vi "BonOMM-SAOMM.vi"() -> ()   [LabVIEW 2019] (continued)
                          frame True {
                            n3695 = Delete From Array(array=w2986, index=0 ("indice")) -> (deleted portion=w2987:string, array with subset deleted=w2985:string[])  [unwired: 1 in]
                            n3696 = case shown="\"MOVE\"" w2987 {
                              tunnel: w2985 -> [_ _ _]
                              frame "", Default {
                              }
                              frame "MOVE" {
                              }
                              frame "STOP" {
                              }
                            }
                          }
                        }
                      }
                      frame "EINF" {
                        n3697 = Decimal String To Number(string=w2990) -> (number=w2991:i32)  [unwired: 2 in, 1 out]
                        n3698 = case shown="1" w2991 {
                          tunnel: [w2995 w3015 "" w3023] -> w2989
                          frame 0, Default {
                            w2996 = "\n"
                            n3699 = Get Date/Time In Seconds() -> (seconds since 1Jan1904=w2994:timestamp)
                            n3700 = local read "Q String"() -> (w2997:string)
                            n3701 = To Double Precision Float(number=w2994) -> (double precision float=w3000:dbl)
                            n3702 = Get Date/Time String(seconds (now)=w3000, want seconds? (F)=TRUE) -> (date string=w2999:string, time string=w2998:string)  [unwired: 1 in]
                            n3703 = Concatenate Strings(w2999, w2996, w2998, w2996, w2997, w2996, "") -> (w2995:string)
                          }
                          frame 1 {
                            w3017 = "Ferme ta yeule, va t'en chez vous! -> "
                            n3704 = local read "Q String"() -> (w3009:string)
                            n3705 = Random Number (0-1)() -> (number: 0 to 1=w3012:dbl)
                            n3706 = Number To Fractional String(number=w3012, precision (6)=i16 12) -> (F-format string=w3010:string)  [unwired: 2 in]
                            n3707 = String Length(string=w3017) -> (length=w3020:i32)
                            n3708 = Number To Decimal String(number=w3020, width (-)=i16 8) -> (decimal integer string=w3018:string)
                            n3709 = Search and Replace String(replace all?=TRUE ("replace all? (F)"), input string=w3009, search string=",", replace string="\r" ("replace string (\"\")")) -> (result string=w3002:string)  [unwired: 4 in, 3 out]
                            n3710 = Concatenate Strings("ANSW", w3018, w3017, w3010) -> (w3014:string)
                            n3711 = Search and Replace String(replace all?=TRUE ("replace all? (F)"), input string=w3002, search string=";", replace string="\r" ("replace string (\"\")")) -> (result string=w3001:string)  [unwired: 4 in, 3 out]
                            n3712 = Select(t=w3001, s=TRUE, f=w3014) -> (s? t:f=w3015:string)
                          }
                          frame 2 {
                          }
                          frame 3 {
                            n3713 = Get Date/Time In Seconds() -> (seconds since 1Jan1904=w3022:timestamp)
                            n3714 = To Double Precision Float(number=w3022) -> (double precision float=w3027:dbl)
                            n3715 = Get Date/Time String(seconds (now)=w3027) -> (date string=w3026:string, time string=w3025:string)  [unwired: 2 in]
                            n3716 = Concatenate Strings(w3026, "\n", w3025) -> (w3023:string)
                          }
                        }
                        n3717 = local write "ANSW"(w2989) -> ()
                      }
                      frame "ECIB" {
                        # "Commande pour retourner le nom et les coordonnées de la cible"
                        n3718 = Decimal String To Number(string=w3029) -> (number=w3030:i32)  [unwired: 2 in, 1 out]
                        n3719 = case shown="1" w3030 {
                          tunnel: [w3034 w3047 "" w3075] -> w3028
                          frame 0, Default {
                            w3035 = "\n"
                            n3720 = Get Date/Time In Seconds() -> (seconds since 1Jan1904=w3033:timestamp)
                            n3721 = local read "Q String"() -> (w3036:string)
                            n3722 = To Double Precision Float(number=w3033) -> (double precision float=w3039:dbl)
                            n3723 = Get Date/Time String(seconds (now)=w3039, want seconds? (F)=TRUE) -> (date string=w3038:string, time string=w3037:string)  [unwired: 1 in]
                            n3724 = Concatenate Strings(w3038, w3035, w3037, w3035, w3036, w3035, "") -> (w3034:string)
                          }
                          frame 1 {
                            w3046 = "0" ("string")
                            w3050 = "\r" ("replace string (\"\")")
                            w3054 = "\r" ("replace string (\"\")")
                            # "Message d'erreur"
                            # "Message contenant les info de la dernière cible chargées"
                            # "Si la coordonnées de la cible est plus loin de 1 degrés de  celle du télescope, on  envoit un message d'erreur"
                            n3725 = local read "Dec_DC"() -> (w3069:string)
                            n3726 = local read "DEC Tel"() -> (w3067:dbl)
                            n3727 = local read "AD_DC"() -> (w3072:string)
                            n3728 = local read "RA Tel"() -> (w3071:dbl)
                            n3729 = Fract/Exp String To Number(string=w3069) -> (number=w3068:dbl)  [unwired: 3 in, 1 out]
                            n3730 = Fract/Exp String To Number(string=w3072) -> (number=w3070:dbl)  [unwired: 3 in, 1 out]
                            n3731 = Divide(x=w3071, y=3600.0) -> (x/y=w3044:dbl)
                            n3732 = Divide(x=w3067, y=3600.0) -> (x/y=w3043:dbl)
                            n3733 = Subtract(x=w3068, y=w3043) -> (x-y=w3065:dbl)
                            n3734 = Subtract(x=w3070, y=w3044) -> (x-y=w3066:dbl)
                            n3735 = Absolute Value(x=w3065) -> (abs(x)=w3064:dbl)
                            n3736 = Absolute Value(x=w3066) -> (abs(x)=w3063:dbl)
                            n3737 = Greater?(x=w3064, y=1.0) -> (0:w3059:bool)
                            n3738 = Greater?(x=w3063, y=0.067) -> (0:w3060:bool)
                            n3739 = local read "DC_button"() -> (w3057:bool)
                            n3740 = Or(x=w3060, y=w3059) -> (x .or. y?=w3058:bool)
                            n3741 = local read "Numero_DC"() -> (w3056:string)
                            n3742 = local read "Nom_DC"() -> (w3055:string)
                            n3743 = local read "Dec_DC"() -> (w3052:string)
                            n3744 = local read "AD_DC"() -> (w3053:string)
                            n3745 = Or(x=w3058, y=w3057) -> (x .or. y?=w3051:bool)
                            n3746 = Not(x=w3051) -> (.not. x?=w3040:bool)
                            n3747 = Concatenate Strings(w3056, w3054, w3055, w3054, w3053, w3054, w3052) -> (w3048:string)
                            n3748 = Concatenate Strings("-1" ("string"), w3050, w3046, w3050, w3046, w3050, w3046) -> (w3049:string)
                            n3749 = Select(t=w3048, s=w3040, f=w3049) -> (s? t:f=w3047:string)
                            n3750 = local write "DC String"(w3047) -> ()
                          }
                          frame 2 {
                          }
                          frame 3 {
                            n3751 = Get Date/Time In Seconds() -> (seconds since 1Jan1904=w3074:timestamp)
                            n3752 = To Double Precision Float(number=w3074) -> (double precision float=w3079:dbl)
                            n3753 = Get Date/Time String(seconds (now)=w3079) -> (date string=w3078:string, time string=w3077:string)  [unwired: 2 in]
                            n3754 = Concatenate Strings(w3078, "\n", w3077) -> (w3075:string)
                          }
                        }
                        n3755 = local write "ANSW"(w3028) -> ()
                      }
                      frame "EAUT" {
                        n3756 = Decimal String To Number(string=w3081) -> (number=w3080:i32)  [unwired: 2 in, 1 out]
                        n3757 = case shown="1, Par défaut" w3080 {
                          frame 1, Default {
                            n3758 = flat-sequence {
                              tunnel: [w3083] -> w3082
                              tunnel: w3082 -> [w3088]
                              frame #0 {
                                n3759 = Two Button Dialog(message="Donnez vous au gouvernement du Québec\nde négocier un entente de parteneriat association  avec le gouvernement du Canada ? \n", 1:"Non" ("F button name (\"Cancel\")"), 2:"Oui" ("T button name (\"OK\")")) -> (T button?=w3083:bool)
                              }
                              frame #1 {
                                n3760 = case shown="Faux" w3088 {
                                tunnel: ["0" "1"] -> w3087
                                frame False {
                                }
                                frame True {
                                }
                                }
                                n3761 = Concatenate Strings(w3087, "\r") -> (w3089:string)
                                n3762 = local write "ANSW"(w3089) -> ()
                              }
                            }
                          }
                        }
                      }
                      frame "ETMP" {
                        n3763 = Decimal String To Number(string=w3094) -> (number=w3093:i32)  [unwired: 2 in, 1 out]
                        n3764 = case shown="1, Par défaut" w3093 {
                          frame 1, Default {
                            w3108 = "\r"
                            n3765 = local read "indic-T-struct"() -> (w3103:dbl)
                            n3766 = local read "indic-H-out"() -> (w3106:dbl)
                            n3767 = local read "indic-H-in"() -> (w3107:dbl)
                            n3768 = local read "indic-T-out"() -> (w3104:dbl)
                            n3769 = local read "indic-T-in"() -> (w3105:dbl)
                            n3770 = local read "indic-Tm"() -> (w3102:dbl)
                            n3771 = Number To Fractional String(number=w3102) -> (F-format string=w3096:string)  [unwired: 3 in]
                            n3772 = Number To Fractional String(number=w3103) -> (F-format string=w3097:string)  [unwired: 3 in]
                            n3773 = Number To Fractional String(number=w3104) -> (F-format string=w3098:string)  [unwired: 3 in]
                            n3774 = Number To Fractional String(number=w3105) -> (F-format string=w3099:string)  [unwired: 3 in]
                            n3775 = Number To Fractional String(number=w3106) -> (F-format string=w3100:string)  [unwired: 3 in]
                            n3776 = Number To Fractional String(number=w3107) -> (F-format string=w3101:string)  [unwired: 3 in]
                            n3777 = Concatenate Strings(w3101, w3108, w3100, w3108, w3099, w3108, w3098, w3108, w3097, w3108, w3096) -> (w3095:string)
                            n3778 = local write "ANSW"(w3095) -> ()
                          }
                        }
                      }
                      frame "EOFF" {
                        n3779 = call "ETAB_decodeur.vi"("chaine entree"=w3110) -> ("Args"=w3111:string[], "nb args"=w3109:u16)  [unwired: 1 out]
                        n3780 = case shown="3" w3109 {
                          tunnel: w3111 -> [_ w3121 w3284]
                          frame 0, Default {
                          }
                          frame 3 {
                            # "Warning Code"
                            # "Error Code"
                            # "Causait erreur\ncode CYGA à modifier"
                            n3781 = Index Array(array=w3121, index #1=0 ("indice"), index #2=1 ("indice"), index #3=2 ("indice")) -> (element #1=w3112:string, element #2=w3115:string, element #3=w3116:string)
                            n3782 = Fract/Exp String To Number(string=w3116) -> (number=w3113:dbl)  [unwired: 3 in, 1 out]
                            n3783 = Fract/Exp String To Number(string=w3115) -> (number=w3114:dbl)  [unwired: 3 in, 1 out]
                            n3784 = stacked-sequence {
                              seq-local: [_ _ w3206 _ _] -> [_ _ _ w3249 _]
                              seq-local: [_ _ w3231 _ _] -> [_ _ _ w3245 _]
                              seq-local: [_ _ w3230 _ _] -> [_ _ _ w3246 _]
                              tunnel: w3113 -> [w3125 w3146 w3212 _ _]
                              tunnel: w3114 -> [w3134 w3145 w3213 _ _]
                              frame #0 {
                                n3785 = local write "Offset RA"(w3134) -> ()
                                n3786 = Number To Fractional String(number=w3134, precision (6)=i16 2) -> (F-format string=w3129:string)  [unwired: 2 in]
                                n3787 = Number To Fractional String(number=w3125, precision (6)=i16 2) -> (F-format string=w3128:string)  [unwired: 2 in]
                                n3788 = local write "Offset DEC"(w3125) -> ()
                                n3789 = local read "Mode Guidage et Dither"() -> (w3123:bool)
                                n3790 = local read "Guidage en cour"() -> (w3124:bool)
                                n3791 = control-ref of="TERMINAL"() -> (w3136:refnum<vi>)
                                n3792 = control-ref of="Indicateur d'état"() -> (w3135:refnum<vi>)
                                n3793 = Concatenate Strings("Envoi externe d'un offset de " ("string"), w3129, ", " ("string"), w3128) -> (w3127:string)
                                n3794 = And(x=w3124, y=w3123) -> (x .and. y?=w3122:bool)
                                n3795 = call "TERMINAL.vi"("Indicateur Refnum"=w3135, "Terminal Refnum"=w3136, "Indicateur d'état"=w3127) -> ()
                                n3796 = case shown="Vrai" w3122 {
                                frame False {
                                }
                                frame True {
                                # "On désactive le guidage et \non indique au code qu'on guidait avant"
                                n3797 = property on="StopServo" class="Bool (strict)"("Val(Sgnl)"=TRUE ("Value (Signaling)")) -> ()  [unwired: 2 in, 2 out]
                                n3798 = local write "StateGuidageDither"(TRUE ("StateGuidageDither")) -> ()
                                }
                                }
                                n3799 = local write "Offset en cours"(TRUE ("enfoncé")) -> ()
                              }
                              frame #1 {
                                # "Si nous somme en train de guider \nEt que lke mode guidage en dither est activé\nAlors bouge le curseur"
                                # "L'échelle est probablement à revoir,\n c'est le ratio pixel/arcsec"
                                n3800 = local read "StateGuidageDither"() -> (w3140:bool)
                                n3801 = local read "Mode Guidage et Dither"() -> (w3139:bool)
                                n3802 = Divide(x=500.0, y=156.0) -> (x/y=w3144:dbl)
                                n3803 = Multiply(x=w3145, y=w3144) -> (x*y=w3143:dbl)
                                n3804 = And(x=w3140, y=w3139) -> (x .and. y?=w3141:bool)
                                n3805 = Multiply(x=w3144, y=w3146) -> (x*y=w3142:dbl)
                                n3806 = case shown="Vrai" w3141 {
                                tunnel: w3143 -> [_ w3151]
                                tunnel: w3142 -> [_ w3150]
                                frame False {
                                }
                                frame True {
                                # "On bouge le curseur de guide \npour s'ajuster au offset"
                                n3807 = Negate(x=w3150) -> (-x=w3149:dbl)
                                n3808 = local read "XReference"() -> (w3152:dbl)
                                n3809 = local read "YReference"() -> (w3153:dbl)
                                n3810 = control-ref of="ImgArray"() -> (w3156:refnum<vi>)
                                n3811 = local read "ROIHeight"() -> (w3158:u16)
                                n3812 = local read "ROIWidth"() -> (w3157:u16)
                                n3813 = Add(x=w3151, y=w3153) -> (x+y=w3155:dbl)
                                n3814 = Add(x=w3149, y=w3152) -> (x+y=w3154:dbl)
                                n3815 = call "SAOMM-Cursor2ROI.vi"("ImgRef"=w3156, "CursorX"=w3154, "CursorY"=w3155, "ROIWidth"=w3157, "ROIHeight"=w3158) -> ("ROIXOffset"=w3159:u16, "ROIYOffset"=w3160:u16)  [unwired: 7 in, 2 out]
                                n3816 = flat-sequence {
                                tunnel: w3159 -> [w3164]
                                tunnel: w3160 -> [w3163]
                                tunnel: [w3164] -> w3162
                                tunnel: [w3163] -> w3161
                                tunnel: w3162 -> [w3170]
                                tunnel: w3161 -> [w3169]
                                frame #0 {
                                n3817 = local write "ROIXOffset"(w3164) -> ()
                                n3818 = local write "ROIYOffset"(w3163) -> ()
                                }
                                frame #1 {
                                n3819 = local read "Binning"() -> (w3190:u16)
                                n3820 = local read "ROIWidth"() -> (w3184:u16)
                                n3821 = local read "ROIHeight"() -> (w3185:u16)
                                n3822 = local read "Naxis1"() -> (w3188:u16)
                                n3823 = local read "Naxis2"() -> (w3187:u16)
                                n3824 = Bundle("ROIXOffset"=w3170, "ROIYOffset"=w3169) -> (w3186:cluster{"ROIXOffset":u16, "ROIYOffset":u16})  [unwired: 1 in]
                                n3825 = local read "XROIRef"() -> (w3182:dbl)
                                n3826 = Bundle("Naxis1"=w3188, "Naxis2"=w3187) -> (w3189:cluster{"Naxis1":u16, "Naxis2":u16})  [unwired: 1 in]
                                n3827 = Bundle("ROIWidth"=w3184, "ROIHeight"=w3185) -> (w3165:cluster{"ROIWidth":u16, "ROIHeight":u16})  [unwired: 1 in]
                                n3828 = local read "YROIRef"() -> (w3168:dbl)
                                n3829 = Bundle("XROIRef"=w3182, "YROIRef"=w3168) -> (w3183:cluster{"XROIRef":dbl, "YROIRef":dbl})  [unwired: 1 in]
                                n3830 = call "SAOMM-ROI_Fixer.vi"("Binning"=w3190, "Use Offset?"=TRUE, "naxis"=w3189, "ROI"=w3165, "Offset"=w3186, "Reference Pixel"=w3183) -> ("FixedOffset"=w3173:cluster{"ROIXOffset":u16, "ROIYOffset":u16}, "FixedPixel"=w3171:cluster{"PixelX":dbl, "PixelY":dbl})  [unwired: 6 in, 2 out]
                                n3831 = Unbundle By Name(w3173) -> ("ROIXOffset"=w3181:u16, "ROIYOffset"=w3180:u16)
                                n3832 = control-ref of="PrAMS-ACK"() -> (w3193:refnum<vi>)
                                n3833 = local read "MessageType"() -> (w3192:cluster{string[], u32[]})
                                n3834 = control-ref of="PrAMS actif"() -> (w3198:refnum<vi>)
                                n3835 = local read "PrAMS VRN"() -> (w3197:refnum<visa-resource-name>)
                                n3836 = local read "PrAMS Error"() -> (w3196:errorcluster)
                                n3837 = Unbundle By Name(w3171) -> ("PixelX"=w3174:dbl, "PixelY"=w3177:dbl)
                                n3838 = To Double Precision Float(number=w3181) -> (double precision float=w3176:dbl)
                                n3839 = To Double Precision Float(number=w3180) -> (double precision float=w3175:dbl)
                                n3840 = Bundle("ROIYOffset"=w3180, "ROIXOffset"=w3181) -> (w3172:cluster{"ROIYOffset":u16, "ROIXOffset":u16})  [unwired: 1 in]
                                n3841 = Add(x=w3175, y=w3174) -> (x+y=w3167:dbl)
                                n3842 = Add(x=w3176, y=w3177) -> (x+y=w3166:dbl)
                                n3843 = call "SAOMM-UpdateROI.vi"("PRAMMS-COMM IN"=w3197, "Active Refnum"=w3198, "PrAMS-ACK"=w3193, "MessageType"=w3192, "Error IN"=w3196, "Position"=w3172) -> ("PRAMMS-COMM OUT"=w3195:refnum<visa-resource-name>, "Error OUT"=w3194:errorcluster)  [unwired: 7 in, 1 out]
                                n3844 = property on="ImgArray" class="GraphInt (strict)"() -> ("Cursor.Cursor Position"=w3179:T45)  [unwired: 2 in, 2 out]
                                n3845 = local write "XReference"(w3167) -> ()
                                n3846 = local write "YReference"(w3166) -> ()
                                n3847 = local write "PrAMS Error"(w3194) -> ()
                                n3848 = local write "PrAMS VRN"(w3195) -> ()
                                n3849 = Bundle(cluster=w3179, "Cursor X"=w3167, "Cursor Y"=w3166) -> (w3178:T45)
                                n3850 = property on="ImgArray" class="GraphInt (strict)"("Cursor.Cursor Position"=w3178) -> ()  [unwired: 2 in, 2 out]
                                }
                                }
                                }
                                }
                              }
                              frame #2 {
                                w3233 = u32 0 ("Error Code IN")
                                n3851 = control-ref of="Mode"() -> (w3214:refnum<vi>)
                                n3852 = control-ref of="Position Z"() -> (w3220:refnum<vi>)
                                n3853 = control-ref of="DiffX"() -> (w3215:refnum<vi>)
                                n3854 = control-ref of="DiffY"() -> (w3216:refnum<vi>)
                                n3855 = control-ref of="SNR"() -> (w3203:refnum<vi>)
                                n3856 = control-ref of="BrasPesto"() -> (w3199:refnum<vi>)
                                n3857 = control-ref of="MovingXY"() -> (w3202:refnum<vi>)
                                n3858 = local read "Table VRN"() -> (w3224:refnum<visa-resource-name>)
                                n3859 = local read "TCS VRN"() -> (w3226:refnum<visa-resource-name>)
                                n3860 = local read "Table Error"() -> (w3223:errorcluster)
                                n3861 = control-ref of="TCS actif"() -> (w3222:refnum<vi>)
                                n3862 = control-ref of="Table actif"() -> (w3221:refnum<vi>)
                                n3863 = control-ref of="StartServo"() -> (w3219:refnum<vi>)
                                n3864 = control-ref of="Servo"() -> (w3218:refnum<vi>)
                                n3865 = control-ref of="StopServo"() -> (w3217:refnum<vi>)
                                n3866 = local read "TCS Error"() -> (w3225:errorcluster)
                                n3867 = control-ref of="LimXPesto"() -> (w3200:refnum<vi>)
                                n3868 = local read "TableAstrom"() -> (w3227:T4)
                                n3869 = local read "FieldAstrom"() -> (w3229:T4)
                                n3870 = local read "GuiderAstrom"() -> (w3228:T4)
                                n3871 = Bundle("TCS VRN"=w3226, "TCS Error"=w3225, "Table VRN"=w3224, "Table Error"=w3223) -> (w3211:T42)  [unwired: 1 in]
                                n3872 = Bundle("TableAstrom"=w3227, "FieldAstrom"=w3229, "GuiderAstrom"=w3228) -> (w3210:T41)  [unwired: 1 in]
                                n3873 = Bundle("TCS actif"=w3222, "Table actif"=w3221, "Position Z"=w3220, "StartServo"=w3219, "Mode"=w3214, "Servo"=w3218, "StopServo"=w3217, "DiffX"=w3215, "DiffY"=w3216, "SNR"=w3203, "MovingXY"=w3202, "BrasPesto"=w3199, "LimXPesto"=w3200) -> (w3209:T43)  [unwired: 1 in]
                                n3874 = call "Cheesy_Offset.vi"("Communications_Cluster"=w3211, "Astrom_Cluster"=w3210, "RA offset"=w3213, "DEC offset"=w3212, "VariablesReferences"=w3209, "OffsetAccuracy (pixels)"="OffsetAcc") -> ("Error code"=w3208:u8, "Undo offset"=w3206:bool, "Warning code"=w3207:u8, "Error Comment"=w3204:string)  [unwired: 6 in]
                                n3875 = while {
                                tunnel: [FALSE] -> w3201
                                stop <- w3240 continue-if-true
                                n3876 = local read "enfoncé"() -> (w3242:bool)
                                n3877 = Not(x=w3242) -> (.not. x?=w3241:bool)
                                n3878 = Wait (ms)(milliseconds to wait=u32 200) -> ()  [unwired: 1 out]
                                n3879 = local write "enfoncé"(w3241) -> ()
                                n3880 = local read "Offset en cours"() -> (w3240:bool)
                                }
                                n3881 = To Unsigned Long Integer(number=w3208) -> (unsigned 32bit integer=w3230:u32)
                                n3882 = To Unsigned Long Integer(number=w3207) -> (unsigned 32bit integer=w3231:u32)
                                n3883 = local read "FIFO d'erreur"() -> (w3234:T7)
                                n3884 = call "Error_Format.vi"("FIFO IN"=w3234, "Error Code IN"=w3233, "Warning Code IN"=w3233, "Error Bit"=w3230, "Warning Bit"=w3231, "Source"="offset", "Comment"=w3204) -> ("FIFO OUT"=w3235:T7)  [unwired: 10 in, 2 out]
                                n3885 = flat-sequence {
                                tunnel: w3235 -> [w3236]
                                frame #0 {
                                n3886 = local write "FIFO d'erreur"(w3236) -> ()
                                }
                                frame #1 {
                                n3887 = local write "Offset en cours"(FALSE) -> ()
                                }
                                }
                                n3888 = local write "enfoncé"(w3201) -> ()
                              }
                              frame #3 {
                                w3251 = FALSE
                                w3244 = FALSE
                                # "Préparation de la réponse ..."
                                n3889 = local write "Offset OK"(w3244) -> ()
                                n3890 = local write "TCS actif"(w3244) -> ()
                                n3891 = local write "RangeTable"(w3251) -> ()
                                n3892 = local write "Calibration"(w3251) -> ()
                                n3893 = local write "stoptable"(w3251) -> ()
                                n3894 = local write "Alacible"(w3251) -> ()
                                n3895 = local write "Origine"(w3251) -> ()
                                n3896 = local write "Centre"(w3251) -> ()
                                n3897 = local read "TERMINAL"() -> (w3255:string)
                                n3898 = Greater Than 0?(x=w3246) -> (x > 0?=w3247:bool)
                                n3899 = case shown="Vrai" w3247 {
                                tunnel: [w3258 w3262] -> w3248
                                tunnel: w3246 -> [_ w3261]
                                tunnel: w3245 -> [w3257 _]
                                frame False {
                                n3900 = Number To Decimal String(number=w3257) -> (decimal integer string=w3260:string)  [unwired: 1 in]
                                n3901 = Concatenate Strings("W" ("string"), w3260) -> (w3258:string)
                                }
                                frame True {
                                n3902 = Number To Decimal String(number=w3261) -> (decimal integer string=w3264:string)  [unwired: 1 in]
                                n3903 = Concatenate Strings("E" ("string"), w3264) -> (w3262:string)
                                }
                                }
                                n3904 = Select(t=" : échoué" ("Command String"), s=w3249, f=" : réussi" ("Command String")) -> (s? t:f=w3256:string)
                                n3905 = Concatenate Strings(w3255, w3256) -> (w3254:string)
                                n3906 = local write "TERMINAL"(w3254) -> ()
                                n3907 = Select(t=w3248, s=w3249, f="OK" ("Command String")) -> (s? t:f=w3243:string)
                                n3908 = local write "ANSW"(w3243) -> ()
                                n3909 = case shown="Vrai" w3249 {
                                frame False {
                                }
                                frame True {
                                n3910 = local read "Table VRN"() -> (w3269:refnum<visa-resource-name>)
                                n3911 = control-ref of="Table actif"() -> (w3267:refnum<vi>)
                                n3912 = local read "Table Error"() -> (w3266:errorcluster)
                                n3913 = control-ref of="TCS actif"() -> (w3270:refnum<vi>)
                                n3914 = local read "TCS VRN"() -> (w3271:refnum<visa-resource-name>)
                                n3915 = call "EXCOM-CMD.vi"("VRN IN"=w3271, "Bool Refnum"=w3270, "Commande #"=13) -> ("VRN OUT"=w3272:refnum<visa-resource-name>, "Error OUT"=w3273:errorcluster)  [unwired: 10 in, 1 out]
                                n3916 = call "Newmark-Stop.vi"("Table VRN IN"=w3269, "Bool Refnum"=w3267, "Error IN"=w3266) -> ("Table VRN OUT"=w3268:refnum<visa-resource-name>, "Error OUT"=w3265:errorcluster)  [unwired: 11 in]
                                n3917 = local write "Table Error"(w3265) -> ()
                                n3918 = local write "Table VRN"(w3268) -> ()
                                n3919 = local write "TCS VRN"(w3272) -> ()
                                n3920 = local write "TCS Error"(w3273) -> ()
                                }
                                }
                              }
                              frame #4 {
                                # "Si le mode de guidage est activé \net qu'on guidait avant"
                                n3921 = local read "StateGuidageDither"() -> (w3275:bool)
                                n3922 = local read "Mode Guidage et Dither"() -> (w3276:bool)
                                n3923 = And(x=w3275, y=w3276) -> (x .and. y?=w3277:bool)
                                n3924 = case shown="Vrai" w3277 {
                                frame False {
                                }
                                frame True {
                                # "Réactive le guidage\nMet la variable de retenir qu'on guidait à off"
                                n3925 = local write "StateGuidageDither"(FALSE ("StateGuidageDither")) -> ()
                                n3926 = property on="StartServo" class="Bool (strict)"("Val(Sgnl)"=TRUE ("Value (Signaling)")) -> ()  [unwired: 2 in, 2 out]
                                }
                                }
                              }
                            }
                            n3927 = Not Equal?(x=w3112, y="N") -> ()  [unwired: 1 out]
                          }
                          frame 4 {
                            # "Lorsqu'il y a un argument additionnel a teloffset."
                            n3928 = Index Array(array=w3284, index #1=0 ("indice"), index #2=1 ("indice"), index #3=2 ("indice"), index #4=3 ("index")) -> (element #1=w3285:string, element #2=w3286:string, element #3=w3287:string, element #4=w3280:string)
                            n3929 = Fract/Exp String To Number(string=w3287) -> (number=w3282:dbl)  [unwired: 3 in, 1 out]
                            n3930 = Fract/Exp String To Number(string=w3286) -> (number=w3283:dbl)  [unwired: 3 in, 1 out]
                            n3931 = Not Equal?(x=w3285, y="N") -> ()  [unwired: 1 out]
                            n3932 = case shown="\"T\"" w3280 {
                              tunnel: w3283 -> [_ w3293]
                              tunnel: w3282 -> [_ w3292]
                              frame "False", Default {
                              }
                              frame "T" {
                                # "Teloffset à l'aide de la télécommande du télescope"
                                n3933 = local write "GE_TCS_RA"(w3293) -> ()
                                n3934 = local write "GE_TCS_DEC"(w3292) -> ()
                              }
                            }
                          }
                        }
                      }
                      frame "ELIB" {
                      }
                      frame "ERAF" {
                        n3935 = call "ETAB_decodeur.vi"("chaine entree"=w3295) -> ("Args"=w3298:string[])  [unwired: 2 out]
                        n3936 = Index Array(array=w3298) -> (element=w3297:string)  [unwired: 1 in]
                        n3937 = local read "MC-BonOMM VRN"() -> (w3296:refnum<visa-resource-name>)
                        n3938 = local read "Excmd VRN"() -> (w3294:refnum<visa-resource-name>)
                        n3939 = case shown="\"i\"" w3297 {
                          selector: w3297 -> [_ _ _ w3337 _]
                          tunnel: w3296 -> [_ w3304 w3320 _ _]
                          tunnel: w3294 -> [_ w3299 w3315 w3334 w3363]
                          frame "", Default {
                          }
                          frame "m" {
                            n3940 = call "MC-BonOMM_talker.vi"("MC-BonOMM VRN"=w3304, "Commande"="m", "byte count"=u32 1, "answer=command?"=FALSE) -> ("Answer"=w3301:string, "ok ?"=w3300:bool)  [unwired: 1 in]
                            n3941 = case shown="Vrai" w3300 {
                              tunnel: w3301 -> [_ w3307]
                              tunnel: w3299 -> [_ w3312]
                              frame False {
                              }
                              frame True {
                                n3942 = Concatenate Strings(w3307, "\n" ("string")) -> (w3306:string)
                                n3943 = String Length(string=w3306) -> (length=w3314:i32)
                                n3944 = Number To Decimal String(number=w3314, width (-)=i16 4 ("largeur (-)")) -> (decimal integer string=w3310:string)
                                n3945 = Concatenate Strings("ANSW", w3310, w3306) -> (w3309:string)
                                n3946 = VISA Write(VISA resource name=w3312, write buffer=w3309) -> ()  [unwired: 1 in, 3 out]
                              }
                            }
                          }
                          frame "q" {
                            n3947 = call "MC-BonOMM_talker.vi"("MC-BonOMM VRN"=w3320, "Commande"="q", "byte count"=u32 1, "answer=command?"=FALSE) -> ("Answer"=w3317:string, "ok ?"=w3316:bool)  [unwired: 1 in]
                            n3948 = case shown="Vrai" w3316 {
                              tunnel: w3317 -> [_ w3324]
                              tunnel: w3315 -> [_ w3328]
                              frame False {
                              }
                              frame True {
                                n3949 = Concatenate Strings(w3324, "\n" ("string")) -> (w3322:string)
                                n3950 = String Length(string=w3322) -> (length=w3330:i32)
                                n3951 = Number To Decimal String(number=w3330, width (-)=i16 4 ("largeur (-)")) -> (decimal integer string=w3326:string)
                                n3952 = Concatenate Strings("ANSW", w3326, w3322) -> (w3325:string)
                                n3953 = VISA Write(VISA resource name=w3328, write buffer=w3325) -> ()  [unwired: 1 in, 3 out]
                              }
                            }
                          }
                          frame "1", "2", "3", "4", "5", "6" {
                            n3954 = Decimal String To Number(string=w3337) -> (number=w3338:i32)  [unwired: 2 in, 1 out]
                            n3955 = case shown="6" w3338 {
                              frame 0, Default {
                              }
                              frame 1 {
                                n3956 = property on="filtre #1" class="Bool (strict)"("Value (Signaling)"=TRUE) -> ()  [unwired: 2 in, 2 out]
                              }
                              frame 2 {
                                n3957 = property on="filtre #2" class="Bool (strict)"("Value (Signaling)"=TRUE) -> ()  [unwired: 2 in, 2 out]
                              }
                              frame 3 {
                                n3958 = property on="filtre #3" class="Bool (strict)"("Value (Signaling)"=TRUE) -> ()  [unwired: 2 in, 2 out]
                              }
                              frame 4 {
                                n3959 = property on="filtre #4" class="Bool (strict)"("Value (Signaling)"=TRUE) -> ()  [unwired: 2 in, 2 out]
                              }
                              frame 5 {
                                n3960 = property on="filtre #5" class="Bool (strict)"("Value (Signaling)"=TRUE) -> ()  [unwired: 2 in, 2 out]
                              }
                              frame 6 {
                                n3961 = property on="filtre #6" class="Bool (strict)"("Value (Signaling)"=TRUE) -> ()  [unwired: 2 in, 2 out]
                              }
                            }
                            n3962 = while {
                              tunnel: w3334 -> [_]
                              tunnel: w3338 -> [w3361]
                              tunnel: [FALSE ("Bypass Tech")] -> w3335
                              tunnel: [w3355] -> w3332
                              tunnel: [w3354] -> w3331
                              i -> [w3359]
                              stop <- w3360 stop-if-true
                              n3963 = local read "F#"() -> (w3355:i32)
                              n3964 = Wait (ms)(milliseconds to wait=u32 200) -> ()  [unwired: 1 out]
                              n3965 = Equal?(x=w3355, y=w3361) -> (x = y?=w3354:bool)
                              n3966 = call "Max-iteration.vi"("i max"=150, "i act"=w3359, "Valeur entrante"=w3354) -> ("break ?"=w3360:bool)
                            }
                            n3967 = Number To Decimal String(number=w3332) -> (decimal integer string=w3333:string)  [unwired: 1 in]
                            n3968 = case shown="Faux" w3331 {
                              tunnel: w3334 -> [_ w3345]
                              tunnel: w3333 -> [_ w3339]
                              frame False {
                              }
                              frame True {
                                n3969 = Concatenate Strings(w3339, "\n" ("string")) -> (w3340:string)
                                n3970 = String Length(string=w3340) -> (length=w3347:i32)
                                n3971 = Number To Decimal String(number=w3347, width (-)=i16 4 ("largeur (-)")) -> (decimal integer string=w3343:string)
                                n3972 = Concatenate Strings("ANSW", w3343, w3340) -> (w3342:string)
                                n3973 = VISA Write(VISA resource name=w3345, write buffer=w3342) -> ()  [unwired: 1 in, 3 out]
                              }
                            }
                            n3974 = local write "Bypass Tech"(w3335) -> ()
                            "Bypass Tech" <- TRUE ("Bypass Tech")
                          }
                          frame "i" {
                            n3975 = local read "Tableau des filtres"() -> (w3370:string[])
                            n3976 = local write "string temporaire"("") -> ()
                            n3977 = for {
                              tunnel: w3370 -> [w3374] mode=indexing
                              tunnel: [w3371] -> w3362
                              n3978 = Concatenate Strings("string temporaire", w3374, "\n" ("string")) -> (w3371:string)
                              n3979 = local write "string temporaire"(w3371) -> ()
                            }
                            n3980 = String Length(string=w3362) -> (length=w3368:i32)
                            n3981 = Number To Decimal String(number=w3368, width (-)=i16 4 ("largeur (-)")) -> (decimal integer string=w3365:string)
                            n3982 = Concatenate Strings("ANSW", w3365, w3362) -> (w3364:string)
                            n3983 = VISA Write(VISA resource name=w3363, write buffer=w3364) -> ()  [unwired: 1 in, 3 out]
                          }
                        }
                      }
                      frame "EHEX" {
                      }
                    }
                  }
                  frame #1 {
                    # "Envoie la réponse sur le port approprié"
                    n3984 = String Subset(string=w3376, length (rest)=3 ("length (rest)")) -> (substring=w3378:string)  [unwired: 1 in]
                    n3985 = Equal?(x=w3378, y="COM") -> (x = y?=w3377:bool)
                    n3986 = case shown="Faux" w3377 {
                      tunnel: w3376 -> [w3391 w3403]
                      tunnel: "ANSW" -> [w3383 w3395]
                      frame False {
                        # "Réponse TCP/IP"
                        n3987 = Type Cast(type=refnum<k5> refnum ("connection ID out"), x=w3391) -> (*(type *) &x=w3390:refnum<k5>)
                        n3988 = String Length(string=w3383) -> (length=w3387:i32)
                        n3989 = Number To Decimal String(number=w3387, width (-)=i16 8) -> (decimal integer string=w3385:string)
                        n3990 = Concatenate Strings("ANSW", w3385, w3383) -> (w3382:string)
                        n3991 = TCP Write(connection ID=w3390, data in=w3382, 9:500 ("timeout ms (25000)")) -> (error out=w3388:errorcluster)  [unwired: 1 in, 2 out]
                        n3992 = local write "TCP/IP Error"(w3388) -> ()
                      }
                      frame True {
                        # "Réponse sur le port Série ..."
                        n3993 = local read "Excmd VRN"() -> (w3404:refnum<visa-resource-name>)
                        n3994 = Type Cast(type=w3404, x=w3403) -> (*(type *) &x=w3402:refnum<visa-resource-name>)
                        n3995 = Concatenate Strings(w3395, "\n") -> (w3396:string)
                        n3996 = String Length(string=w3396) -> (length=w3400:i32)
                        n3997 = Number To Decimal String(number=w3400, width (-)=i16 4) -> (decimal integer string=w3399:string)
                        n3998 = Concatenate Strings("ANSW", w3399, w3396) -> (w3397:string)
                        n3999 = local read "Excom Error"() -> (w3393:errorcluster)
                        n4000 = VISA Write(VISA resource name=w3402, write buffer=w3397, error in (no error)=w3393) -> (error out=w3392:errorcluster)  [unwired: 2 out]
                        n4001 = local write "Excom Error"(w3392) -> ()
                      }
                    }
                  }
                }
                "Error Code" <- w2858
                "Warning Code" <- w2858
              }
            }
            n4002 = Wait Until Next ms Multiple(millisecond multiple=u32 50 ("n millisecondes")) -> ()  [unwired: 1 out]
            n4003 = local read "Quit"() -> (w2851:bool)
          }
          "Gestion Scripts" <- w970
          n4004 = while {
            tunnel: [w1440] -> w975
            i -> [w1441]
            stop <- w1440 stop-if-true
            n4005 = event shown="[0] Timeout" {
              selector: _ -> [_ _ _ _ _ _ _ _ _ _ _ _ _ _ _ _ _ _ _ _ _ _ _]
              dyn-events: _ -> [_ _ _ _ _ _ _ _ _ _ _ _ _ _ _ _ _ _ _ _ _ _ _]
              timeout: 200 -> [_ _ _ _ _ _ _ _ _ _ _ _ _ _ _ _ _ _ _ _ _ _ _]
              tunnel: w1441 -> [w1449 _ _ _ _ _ _ _ _ _ _ _ _ _ _ _ _ _ _ _ _ _ _]
              event Timeout {
                # "À passer dans une boucle à part ?"
                n4006 = event-data() -> ()  [unwired: 1 in, 2 out]
                n4007 = local read "Integrating"() -> (w1446:bool)
                n4008 = Quotient & Remainder(x=w1449, y=25) -> (x-y*floor(x/y)=w1447:i32)  [unwired: 1 out]
                n4009 = Equal To 0?(x=w1449) -> (x = 0?=w1451:bool)
                n4010 = Equal To 0?(x=w1447) -> (x = 0?=w1445:bool)
                n4011 = Not(x=w1446) -> (.not. x?=w1444:bool)
                n4012 = And(x=w1445, y=w1444) -> (x .and. y?=w1443:bool)
                n4013 = Or(x="FalconRefresh", y=w1451) -> (x .or. y?=w1456:bool)
                n4014 = Equal?(x=w1449, y=1) -> (x = y?=w1453:bool)
                n4015 = Compound Arithmetic op=OR(w1453, "HexapodRefresh", w1443) -> (w1450:bool)
                n4016 = case shown="Faux" w1456 {
                  frame False {
                  }
                  frame True {
                    n4017 = Tick Count (ms)() -> (millisecond timer value=→"FalconQuery":u32)
                    n4018 = local write "FalconRefresh"(FALSE ("Refresh")) -> ()
                    n4019 = local read "PrAMS VRN"() -> (w1473:refnum<visa-resource-name>)
                    n4020 = local read "PrAMS Error"() -> (w1475:errorcluster)
                    n4021 = local read "MessageType"() -> (w1470:cluster{string[], u32[]})
                    n4022 = control-ref of="PrAMS actif"() -> (w1471:refnum<vi>)
                    n4023 = local read "Signature"() -> (w1469:u32)
                    n4024 = call "SAOMM-QueryFalcon.vi"("PRAMMS-COMM IN"=w1473, "Bool Refnum"=w1471, "Signature"=w1469, "Error IN"=w1475, "CommandCluster"=w1470) -> ("PRAMMS-COMM OUT"=w1472:refnum<visa-resource-name>, "Error OUT"=w1474:errorcluster)  [unwired: 9 in]
                    n4025 = local write "PrAMS Error"(w1474) -> ()
                    n4026 = local write "PrAMS VRN"(w1472) -> ()
                    "QueryingPraMS" <- TRUE
                  }
                }
                n4027 = case shown="Vrai" w1450 {
                  frame False {
                  }
                  frame True {
                    n4028 = local write "HexapodRefresh"(FALSE ("Refresh")) -> ()
                    n4029 = Tick Count (ms)() -> (millisecond timer value=→"HexapodQuery":u32)
                    n4030 = local read "MessageType"() -> (w1462:cluster{string[], u32[]})
                    n4031 = control-ref of="HexaCons actif"() -> (w1458:refnum<vi>)
                    n4032 = local read "PrAMS Error"() -> (w1464:errorcluster)
                    n4033 = local read "Signature"() -> (w1461:u32)
                    n4034 = call "SAOMM-QueryHexapod.vi"("PRAMMS-COMM IN"="Hexapod VRN", "Bool Refnum"=w1458, "Signature"=w1461, "Error IN"=w1464, "EnumMessageType"=w1462) -> ("PRAMMS-COMM OUT"=w1459:refnum<visa-resource-name>, "Error OUT"=w1463:errorcluster)  [unwired: 9 in]
                    n4035 = local write "PrAMS Error"(w1463) -> ()
                    n4036 = local write "Hexapod VRN"(w1459) -> ()
                    "QueryingHexapod" <- TRUE ("Refresh")
                  }
                }
              }
              event "refresh": Value Change {
                n4037 = event-data() -> ()  [unwired: 1 in, 5 out]
                n4038 = case shown="Vrai" "refresh" {
                  frame False {
                  }
                  frame True {
                    n4039 = flat-sequence {
                      frame #0 {
                        n4040 = local read "MessageType"() -> (w1485:cluster{string[], u32[]})
                        n4041 = control-ref of="PrAMS actif"() -> (w1484:refnum<vi>)
                        n4042 = local read "PrAMS VRN"() -> (w1483:refnum<visa-resource-name>)
                        n4043 = local read "PrAMS Error"() -> (w1482:errorcluster)
                        n4044 = local read "Signature"() -> (w1481:u32)
                        n4045 = call "SAOMM-SendGET.vi"("PRAMMS-COMM IN"=w1483, "Bool Refnum"=w1484, "MessageType"=w1485, "Signature"=w1481, "Error IN"=w1482, "Active GET"="GetCommand") -> ("PRAMMS-COMM OUT"=w1480:refnum<visa-resource-name>, "Error OUT"=w1479:errorcluster)  [unwired: 8 in]
                        n4046 = local write "PrAMS Error"(w1479) -> ()
                        n4047 = local write "PrAMS VRN"(w1480) -> ()
                      }
                      frame #1 {
                        n4048 = local write "refresh"(FALSE) -> ()
                      }
                    }
                  }
                }
              }
              event "Mode": Value Change {
                # "C'est ici qu'on changera les mutex pour les boutons quand ceux-ci seront définis ..."
                n4049 = event-data() -> ("OldVal"=w1488:u16, "NewVal"=w1487:u16)  [unwired: 1 in, 3 out]
                n4050 = case shown="0, Par défaut" w1488 {
                  frame 0, Default {
                    # "On passe de 'Opération fixe' à ..."
                  }
                  frame 1 {
                    # "On passe de 'Asservissement passif' à ..."
                  }
                  frame 2 {
                    # "On passe de 'Asservissement actif' à ..."
                  }
                  frame 3 {
                    # "On passe de 'Calibration' à ..."
                  }
                }
                n4051 = case shown="1..3" w1487 {
                  frame 0, Default {
                    # "... 'Opération fixe'"
                  }
                  frame 4 {
                    w1489 = T17."Enabled" ("Disabled")
                    # "On passe de 'Opération fixe' à ..."
                    n4052 = property on="StartServo" class="Bool (strict)"("DisabledEnum"=w1489) -> ()  [unwired: 2 in, 2 out]
                    n4053 = property on="StopServo" class="Bool (strict)"("DisabledEnum"=w1489) -> ()  [unwired: 2 in, 2 out]
                  }
                  frame 1..3 {
                    # "'Asservissement passif'"
                    n4054 = local read "Integrating"() -> (w1490:bool)
                    n4055 = case shown="Faux" w1490 {
                      frame False {
                        w1491 = T17."Disabled and Grayed Out" ("Disabled")
                        n4056 = property on="StopServo" class="Bool (strict)"("DisabledEnum"=w1491) -> ()  [unwired: 2 in, 2 out]
                        n4057 = property on="StartServo" class="Bool (strict)"("DisabledEnum"=w1491) -> ()  [unwired: 2 in, 2 out]
                      }
                      frame True {
                      }
                    }
                  }
                }
              }
              event "ImgArray": Mouse Down {
                n4058 = event-data() -> ("Coords"=w1496:T50)  [unwired: 1 in, 6 out]
                n4059 = local read "Integrating"() -> (w1494:bool)
                n4060 = local read "Servo"() -> (w1493:bool)
                n4061 = Not(x=w1493) -> (.not. x?=w1492:bool)
                n4062 = And(x=w1494, y=w1492) -> (x .and. y?=w1495:bool)
                n4063 = case shown="Vrai" w1495 {
                  tunnel: w1496 -> [_ w1531]
                  tunnel: w1492 -> [w1497 _]
                  frame False {
                    n4064 = case shown="Faux" w1497 {
                      frame False {
                        n4065 = One Button Dialog(message="Vous ne pouvez pas modifier la ROI pendant l'asservissement") -> ()  [unwired: 1 in, 1 out]
                      }
                      frame True {
                      }
                    }
                  }
                  frame True {
                    n4066 = control-ref of="ImgArray"() -> (w1528:refnum<vi>)
                    n4067 = local read "ROIWidth"() -> (w1527:u16)
                    n4068 = local read "ROIHeight"() -> (w1526:u16)
                    n4069 = call "Click2CursorPosition.vi"("reference"=w1528, "ClickPosition"=w1531) -> ("CursorX"=w1530:dbl, "CursorY"=w1529:dbl)  [unwired: 12 in]
                    n4070 = call "SAOMM-Cursor2ROI.vi"("ImgRef"=w1528, "CursorX"=w1530, "CursorY"=w1529, "ROIWidth"=w1527, "ROIHeight"=w1526) -> ("XÉtoile"=w1504:dbl, "YÉtoile"=w1503:dbl, "ROIXOffset"=w1508:u16, "ROIYOffset"=w1507:u16)  [unwired: 7 in]
                    n4071 = local write "YROIRef"(w1504) -> ()
                    n4072 = local write "XROIRef"(w1503) -> ()
                    n4073 = local write "ROIXOffset"(w1508) -> ()
                    n4074 = local write "ROIYOffset"(w1507) -> ()
                    n4075 = local read "Binning"() -> (w1517:u16)
                    n4076 = local read "ROIWidth"() -> (w1510:u16)
                    n4077 = local read "ROIHeight"() -> (w1511:u16)
                    n4078 = local read "Naxis1"() -> (w1515:u16)
                    n4079 = local read "Naxis2"() -> (w1514:u16)
                    n4080 = Bundle("XÉtoile"=w1504, "YÉtoile"=w1503) -> (w1509:cluster{"XÉtoile":dbl, "YÉtoile":dbl})  [unwired: 1 in]
                    n4081 = Bundle("Naxis1"=w1515, "Naxis2"=w1514) -> (w1516:cluster{"Naxis1":u16, "Naxis2":u16})  [unwired: 1 in]
                    n4082 = Bundle("ROIWidth"=w1510, "ROIHeight"=w1511) -> (w1513:cluster{"ROIWidth":u16, "ROIHeight":u16})  [unwired: 1 in]
                    n4083 = Bundle("ROIXOffset"=w1508, "ROIYOffset"=w1507) -> (w1512:cluster{"ROIXOffset":u16, "ROIYOffset":u16})  [unwired: 1 in]
                    n4084 = control-ref of="PrAMS-ACK"() -> (w1520:refnum<vi>)
                    n4085 = local read "MessageType"() -> (w1519:cluster{string[], u32[]})
                    n4086 = control-ref of="PrAMS actif"() -> (w1525:refnum<vi>)
                    n4087 = local read "PrAMS VRN"() -> (w1524:refnum<visa-resource-name>)
                    n4088 = local read "PrAMS Error"() -> (w1523:errorcluster)
                    n4089 = call "SAOMM-ROI_Fixer.vi"("Binning"=w1517, "Use Offset?"=TRUE, "naxis"=w1516, "ROI"=w1513, "Offset"=w1512, "Reference Pixel"=w1509) -> ("FixedOffset"=w1501:cluster{"ROIXOffset":u16, "ROIYOffset":u16}, "FixedPixel"=w1502:cluster{"PixelX":dbl, "PixelY":dbl})  [unwired: 6 in, 2 out]
                    n4090 = Unbundle By Name(w1502) -> ("PixelX"=w1500:dbl, "PixelY"=w1499:dbl)
                    n4091 = call "SAOMM-UpdateROI.vi"("PRAMMS-COMM IN"=w1524, "Active Refnum"=w1525, "PrAMS-ACK"=w1520, "MessageType"=w1519, "Error IN"=w1523, "Position"=w1501) -> ("PRAMMS-COMM OUT"=w1522:refnum<visa-resource-name>, "Error OUT"=w1521:errorcluster)  [unwired: 7 in, 1 out]
                    n4092 = local write "PrAMS Error"(w1521) -> ()
                    n4093 = local write "PrAMS VRN"(w1522) -> ()
                    n4094 = property on="ImgArray" class="GraphInt (strict)"() -> ("Cursor.Cursor Position"=w1506:T45)  [unwired: 2 in, 2 out]
                    n4095 = local write "XReference"(w1500) -> ()
                    n4096 = local write "YReference"(w1499) -> ()
                    n4097 = Bundle(cluster=w1506, "Cursor X"=w1500, "Cursor Y"=w1499) -> (w1505:T45)
                    n4098 = property on="ImgArray" class="GraphInt (strict)"("Cursor.Cursor Position"=w1505) -> ()  [unwired: 2 in, 2 out]
                  }
                }
              }
              event "ClearDump": Value Change {
                # "Tout ceci est du débuggage ..."
                n4099 = event-data() -> ()  [unwired: 1 in, 5 out]
                n4100 = local write "nDumped"(0 ("nDumped")) -> ()
                n4101 = local write "Dump"("") -> ()
              }
              event "ImageFPS": Value Change {
                n4102 = event-data() -> ()  [unwired: 1 in, 5 out]
                n4103 = flat-sequence {
                  tunnel: [w1536] -> w1535
                  tunnel: [w1539] -> w1534
                  tunnel: w1535 -> [w1539]
                  tunnel: w1534 -> [w1551]
                  frame #0 {
                    n4104 = Tick Count (ms)() -> (millisecond timer value=w1536:u32)
                  }
                  frame #1 {
                    n4105 = local read "MessageType"() -> (w1542:cluster{string[], u32[]})
                    n4106 = control-ref of="PrAMS-ACK"() -> (w1543:refnum<vi>)
                    n4107 = control-ref of="PrAMS actif"() -> (w1544:refnum<vi>)
                    n4108 = local read "PrAMS Error"() -> (w1545:errorcluster)
                    n4109 = local read "PrAMS VRN"() -> (w1546:refnum<visa-resource-name>)
                    n4110 = local read "ImageFPS"() -> (w1537:dbl)
                    n4111 = local read "Signature"() -> (w1538:u32)
                    n4112 = call-poly "SAOMM-Num2littleEndian.vi"("Number"=w1537) -> ("LiitleEndianedData"=w1540:u8[])  [unwired: 14 in]
                    n4113 = call "SAOMM-SendSET.vi"("PRAMMS-COMM IN"=w1546, "Active Refnum"=w1544, "PrAMS-ACK"=w1543, "Signature"=w1538, "Error IN"=w1545, "MessageType"=w1542, "Active SET"="emtSetImageDisplayFrameRate", "Value (little endianed byte array)"=w1540) -> ("PRAMMS-COMM OUT"=w1548:refnum<visa-resource-name>, "Error OUT"=w1547:errorcluster)  [unwired: 4 in, 2 out]
                    n4114 = local write "PrAMS Error"(w1547) -> ()
                    n4115 = local write "PrAMS VRN"(w1548) -> ()
                  }
                  frame #2 {
                    n4116 = Tick Count (ms)() -> (millisecond timer value=w1550:u32)
                    n4117 = Subtract(x=w1550, y=w1551) -> (x-y=→"SetFPSTime":u32)
                  }
                }
              }
              event "exptime": Value Change {
                n4118 = event-data() -> ()  [unwired: 1 in, 5 out]
                n4119 = flat-sequence {
                  tunnel: [w1554] -> w1553
                  tunnel: [w1556] -> w1552
                  tunnel: w1553 -> [w1556]
                  tunnel: w1552 -> [w1571]
                  frame #0 {
                    n4120 = Tick Count (ms)() -> (millisecond timer value=w1554:u32)
                  }
                  frame #1 {
                    n4121 = local read "MessageType"() -> (w1562:cluster{string[], u32[]})
                    n4122 = control-ref of="PrAMS-ACK"() -> (w1563:refnum<vi>)
                    n4123 = control-ref of="PrAMS actif"() -> (w1564:refnum<vi>)
                    n4124 = local read "PrAMS Error"() -> (w1565:errorcluster)
                    n4125 = local read "PrAMS VRN"() -> (w1566:refnum<visa-resource-name>)
                    n4126 = expression code="x*1000"("exptime") -> (w1558:dbl)
                    n4127 = local read "Signature"() -> (w1555:u32)
                    n4128 = To Unsigned Long Integer(number=w1558) -> (unsigned 32bit integer=w1557:u32)
                    n4129 = call-poly "SAOMM-Num2littleEndian.vi"("Number"=w1557) -> ("LiitleEndianedData"=w1560:u8[])  [unwired: 14 in]
                    n4130 = call "SAOMM-SendSET.vi"("PRAMMS-COMM IN"=w1566, "Active Refnum"=w1564, "PrAMS-ACK"=w1563, "Signature"=w1555, "Error IN"=w1565, "MessageType"=w1562, "Active SET"="emtSetImageExposureTime", "Value (little endianed byte array)"=w1560) -> ("PRAMMS-COMM OUT"=w1568:refnum<visa-resource-name>, "Error OUT"=w1567:errorcluster)  [unwired: 4 in, 2 out]
                    n4131 = local write "PrAMS Error"(w1567) -> ()
                    n4132 = local write "PrAMS VRN"(w1568) -> ()
                  }
                  frame #2 {
                    n4133 = Tick Count (ms)() -> (millisecond timer value=w1570:u32)
                    n4134 = Subtract(x=w1570, y=w1571) -> (x-y=→"SetExpTime":u32)
                  }
                }
              }
              event "FPGA Value": Value Change {
                n4135 = event-data() -> ("NewVal"=w1575:u16)  [unwired: 1 in, 4 out]
                n4136 = local read "Integrating"() -> (w1572:bool)
                n4137 = local read "Servo"() -> (w1573:bool)
                n4138 = Or(x=w1573, y=w1572) -> (x .or. y?=w1574:bool)
                n4139 = case shown="Faux" w1574 {
                  tunnel: w1575 -> [w1580 _]
                  frame False {
                    n4140 = Number To Decimal String(number=w1580) -> (decimal integer string=w1579:string)  [unwired: 1 in]
                    n4141 = call-poly "SAOMM-Num2littleEndian.vi"("Number"=w1580) -> ("LiitleEndianedData"=w1583:u8[])  [unwired: 14 in]
                    n4142 = local read "MessageType"() -> (w1586:cluster{string[], u32[]})
                    n4143 = control-ref of="PrAMS-ACK"() -> (w1587:refnum<vi>)
                    n4144 = control-ref of="PrAMS actif"() -> (w1588:refnum<vi>)
                    n4145 = local read "PrAMS VRN"() -> (w1590:refnum<visa-resource-name>)
                    n4146 = local read "PrAMS Error"() -> (w1589:errorcluster)
                    n4147 = control-ref of="TERMINAL"() -> (w1581:refnum<vi>)
                    n4148 = control-ref of="Indicateur d'état"() -> (w1582:refnum<vi>)
                    n4149 = local read "Signature"() -> (w1584:u32)
